vi "libssh2_channel_read.vi"(8 "error in (no error)":errorcluster, 10 "buffer length":i32=1024, 11 "channel":T1) -> (0 "error out":errorcluster, 2 "buffer":u8[](array[numeric]))   [LabVIEW 2013, in "libssh2.lvlib"]
doc: "Reads data from the standard I/O substream."
uses:
  libssh2.lvlib
  Channel Refnum.ctl
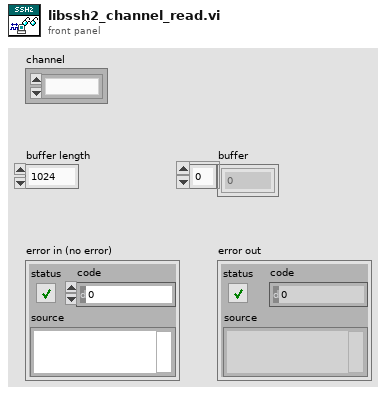
[diagram p1: front panel]
types:
  T1 = typedef "libssh2.lvlib/Channel Refnum.ctl" = refnum<k1>
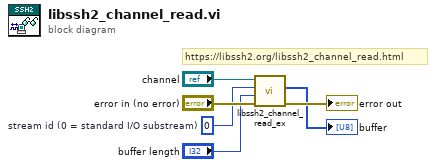
[diagram p0: block diagram]
diagram:
  w1 = 0  # stream id (0 = standard I/O substream)
  # "https://libssh2.org/libssh2_channel_read.html"
  n1 = call "libssh2_channel_read_ex.vi"("error in (no error)"="error in (no error)", "buffer length"="buffer length", "stream id"=w1, "channel"="channel") -> ("error out"=→"error out":errorcluster, "buffer"=→"buffer":u8[])  [unwired: 6 in]
